vi "Condition _string_4_REJECTION.vi"(0 "From Date":timestamp format="%<%Y-%m-%d>T", 1 "Select Stakeholder":string(combo), 5 "To Date":timestamp format="%<%Y-%m-%d>T", 7 "Shift":string(combo)="ALL", 9 "Select Station":string(combo)="ST 1", 11 "STACKHOLDER_ID":i32, 12 "Refnum out 2":T1) -> (3 "Array":string[](array[string]), 4 "sum":i32[](array[numeric]), 6 "all station":string[][](array[string]), 8 "Table":string[][](array[string]), 10 "Elements Found out":string[](array[string]), 13 "PROD_COUNT TEST":string[](array[string]), 14 "Refnum out":T1, 15 "Array 3":string[][](array[string]))   [LabVIEW 2017]
uses:
  <vilib>/addons/database/Connection.llb/Conn ObjectReference.ctl
  <vilib>/addons/database/NI_Database_API.lvlib
panel:
  out "COUNT":string[](array[string])
  out "DATE":string[](array[string])
  out "error out":errorcluster
  in  "error in (no error)":errorcluster
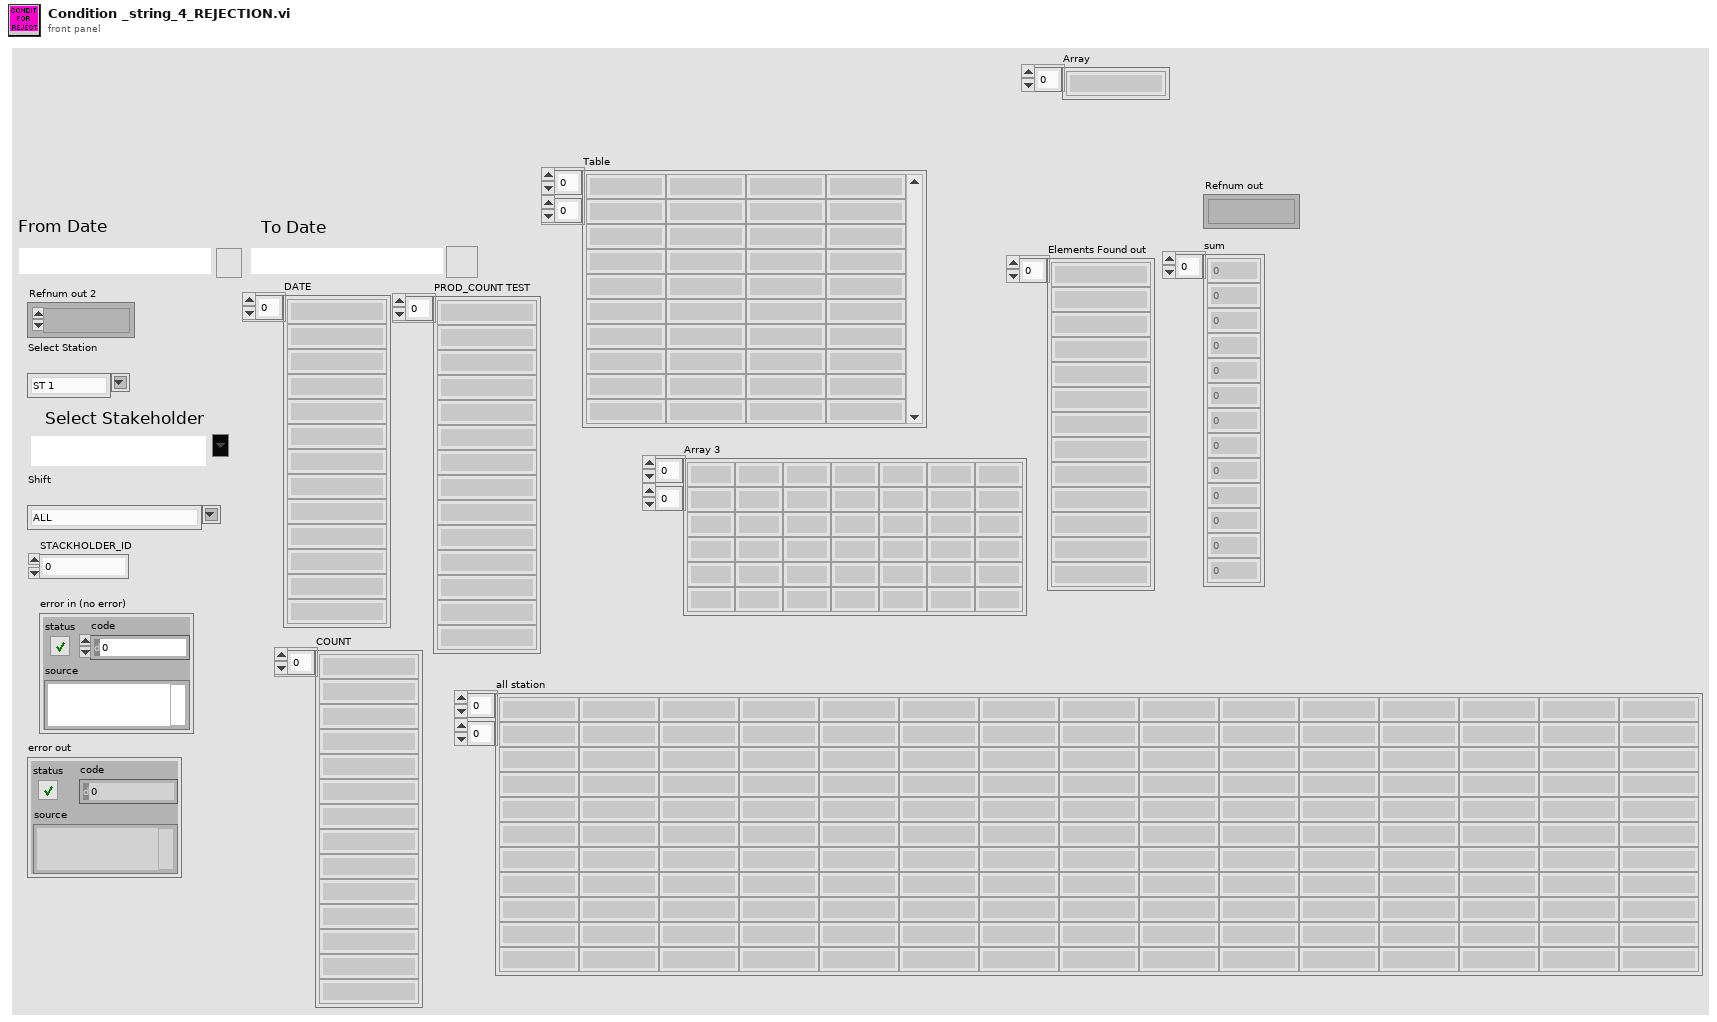
[diagram p1: front panel]
types:
  T1 = typedef "NI_Database_API.lvlib/Conn ObjectReference.ctl" = refnum<k1>
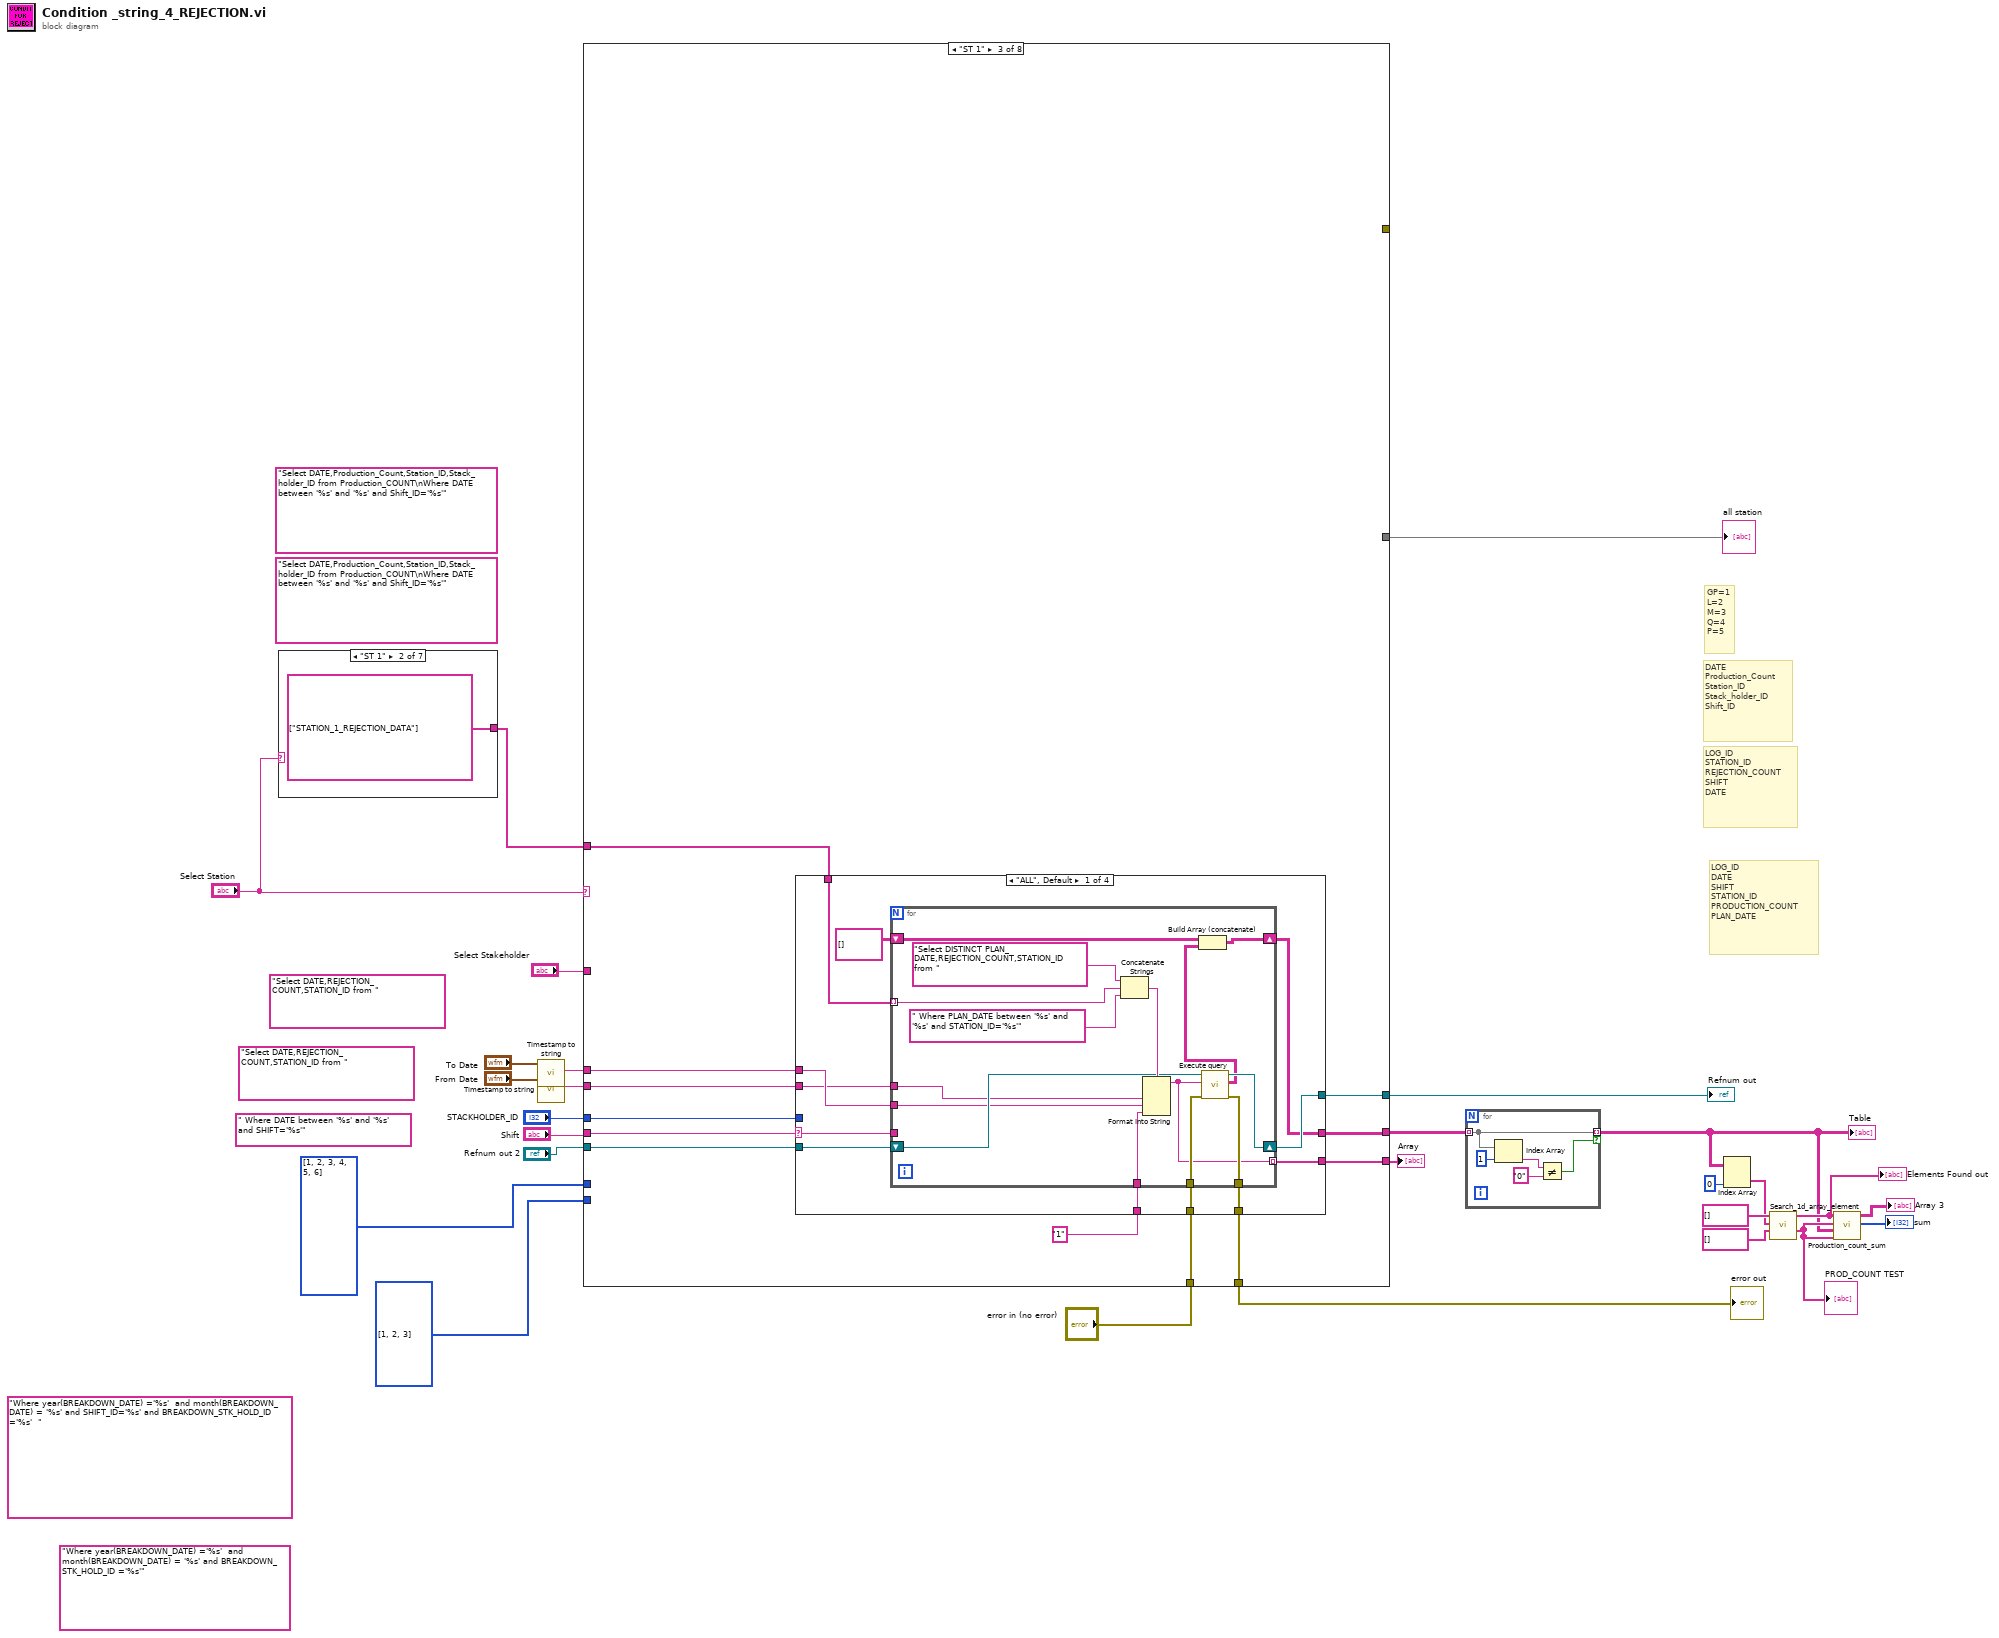
[diagram p0: block diagram]
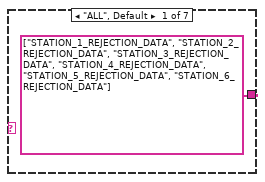
[diagram p2: hidden frame]
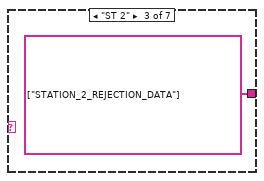
[diagram p3: hidden frame]
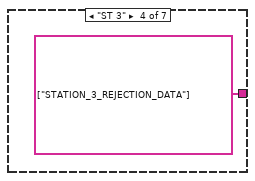
[diagram p4: hidden frame]
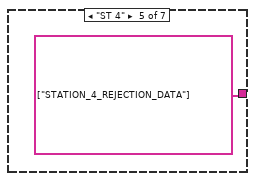
[diagram p5: hidden frame]
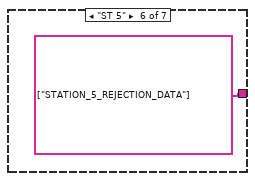
[diagram p6: hidden frame]
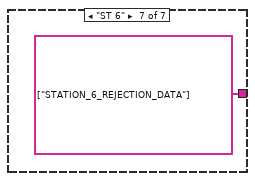
[diagram p7: hidden frame]
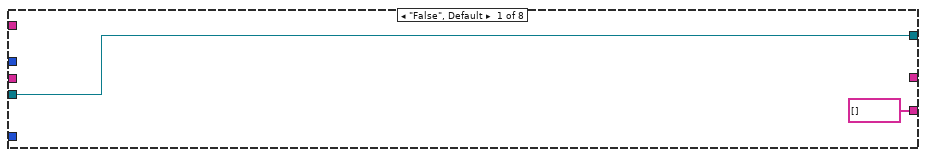
[diagram p8: hidden frame]
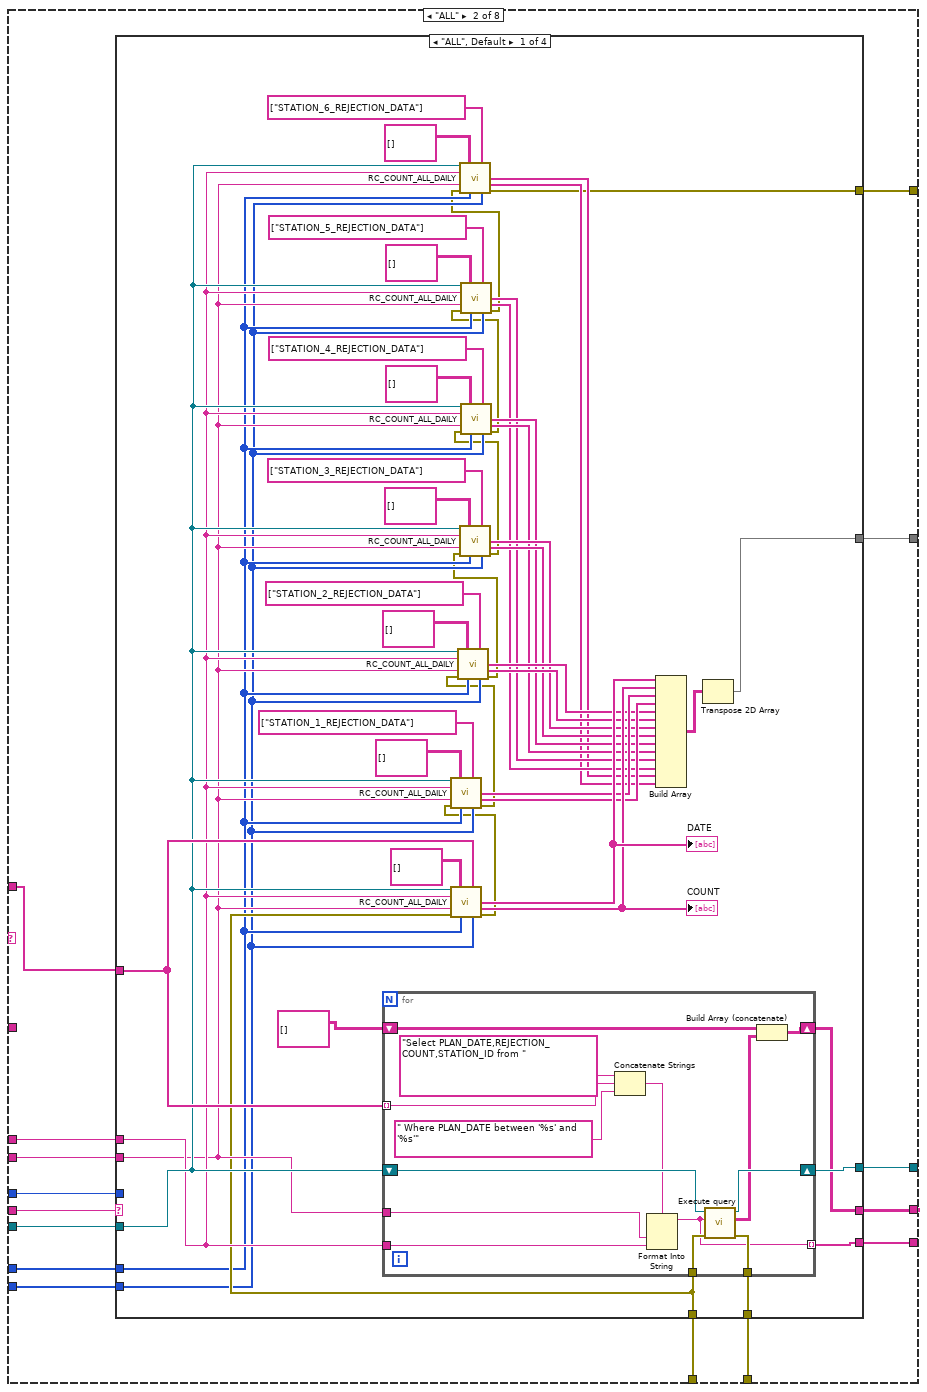
[diagram p9: hidden frame]
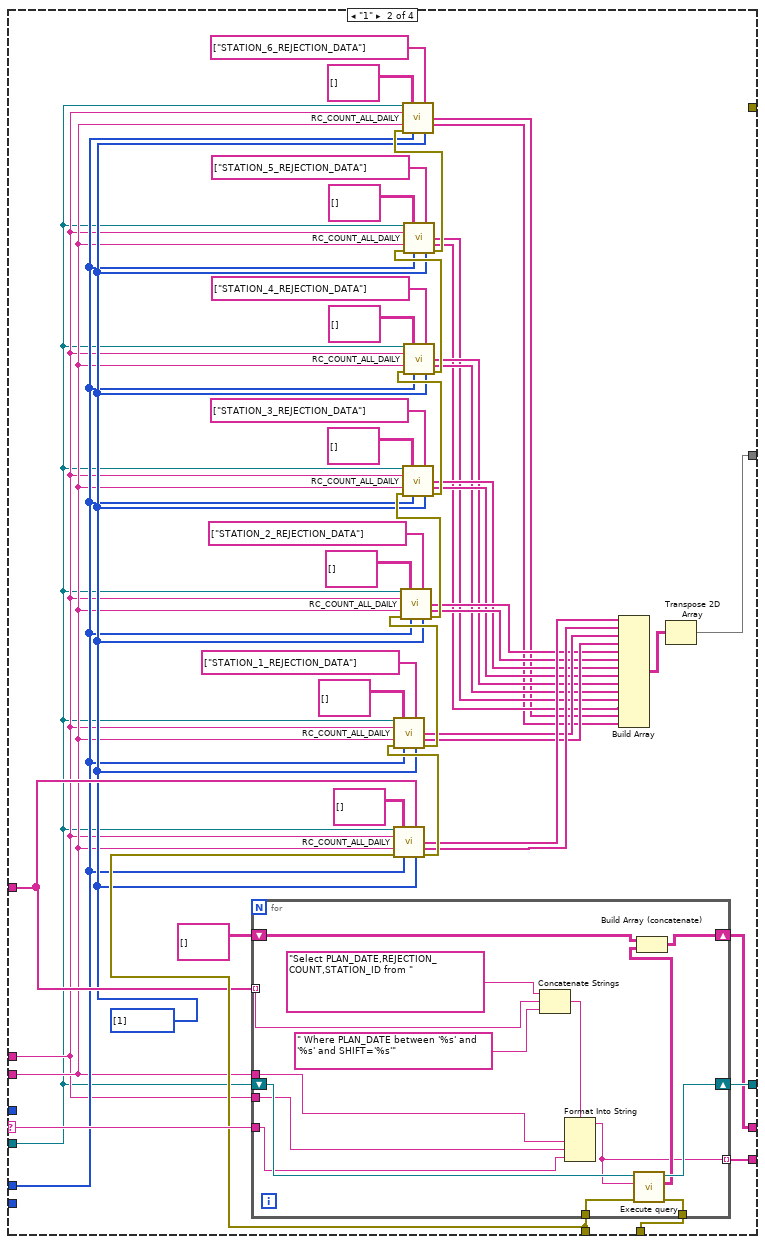
[diagram p10: hidden frame]
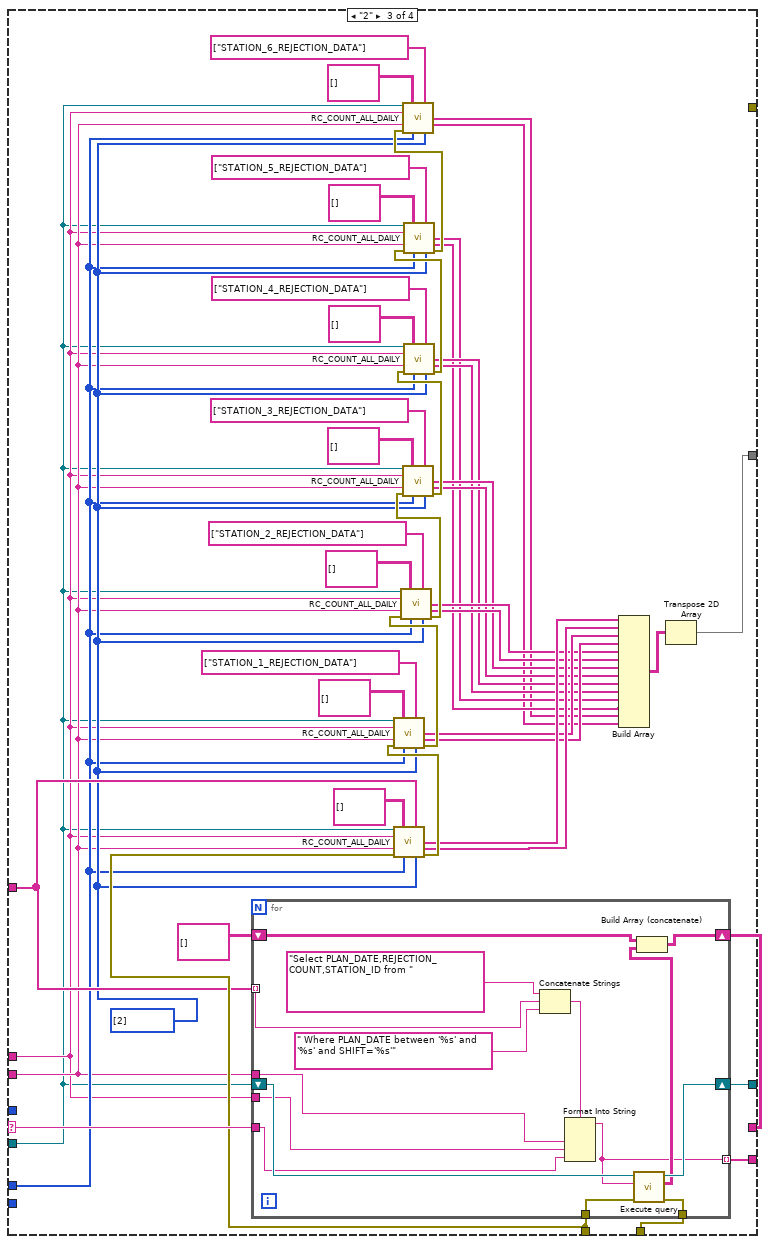
[diagram p11: hidden frame]
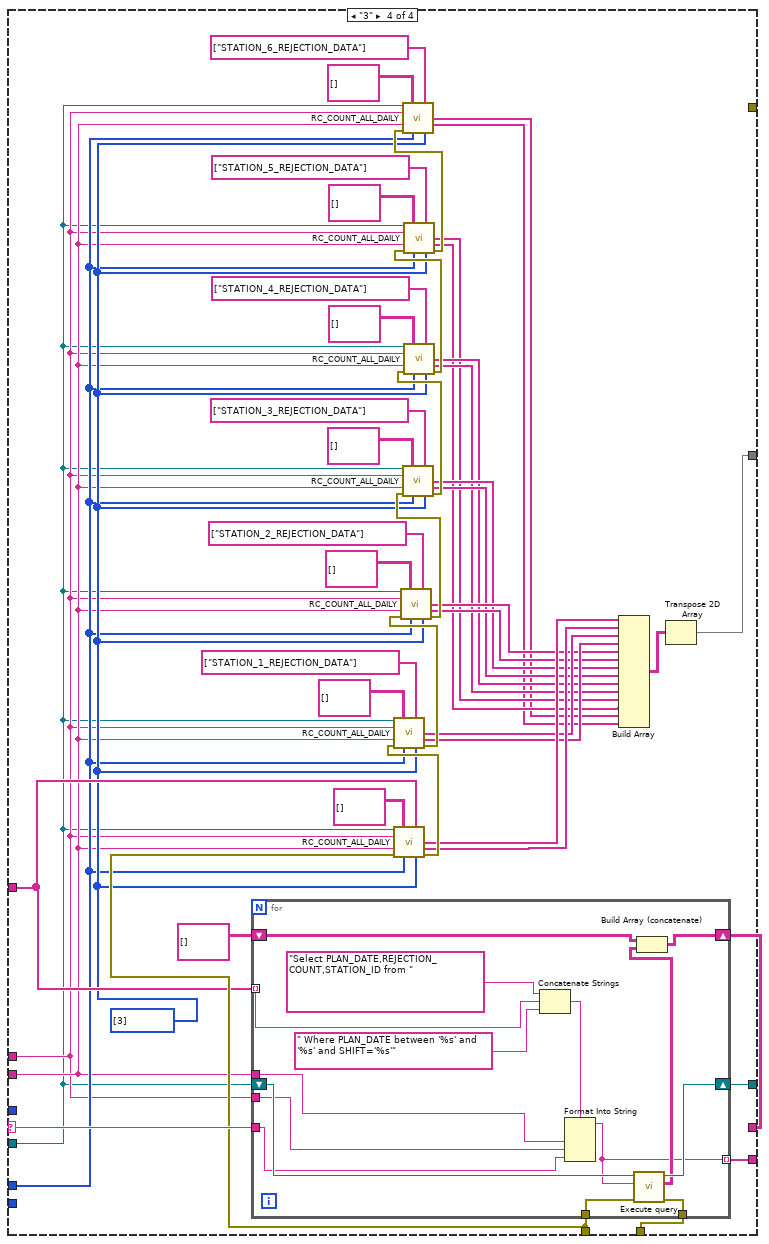
[diagram p12: hidden frame]
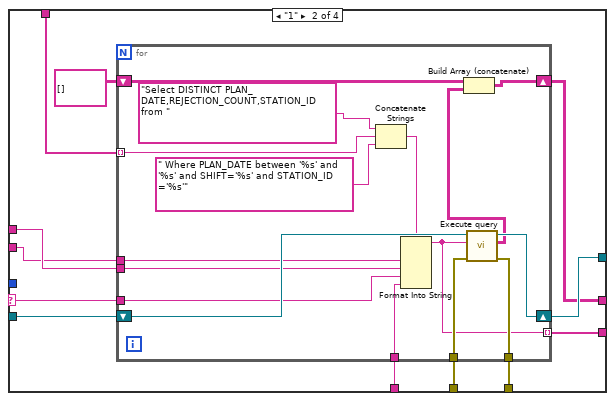
[diagram p13: hidden frame]
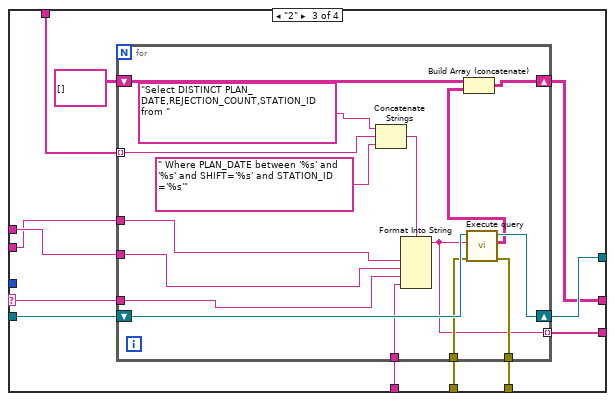
[diagram p14: hidden frame]
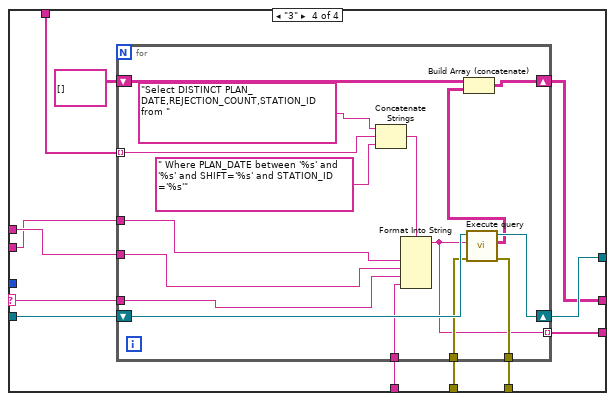
[diagram p15: hidden frame]
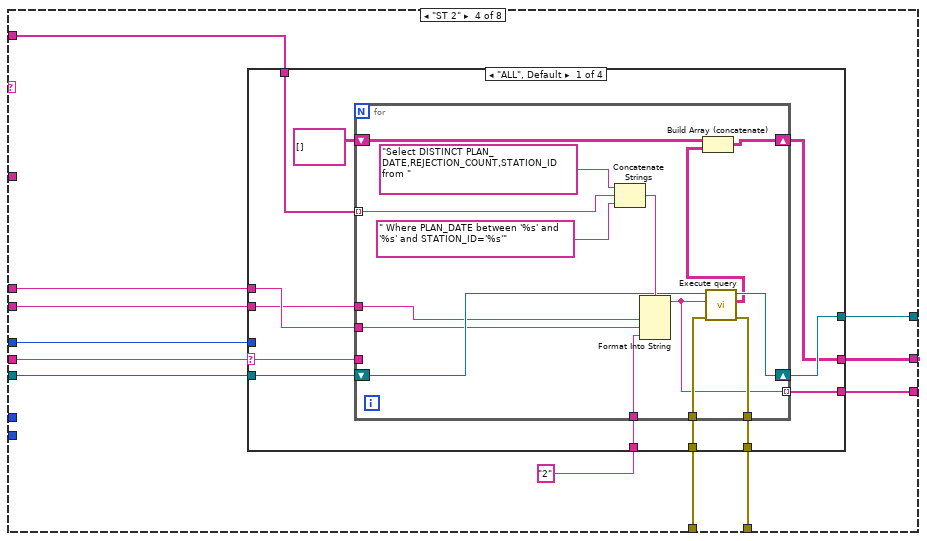
[diagram p16: hidden frame]
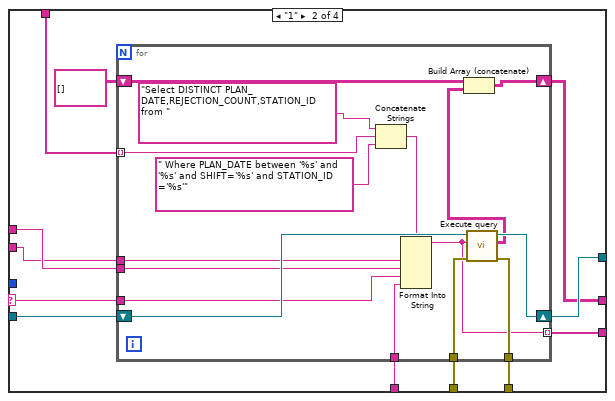
[diagram p17: hidden frame]
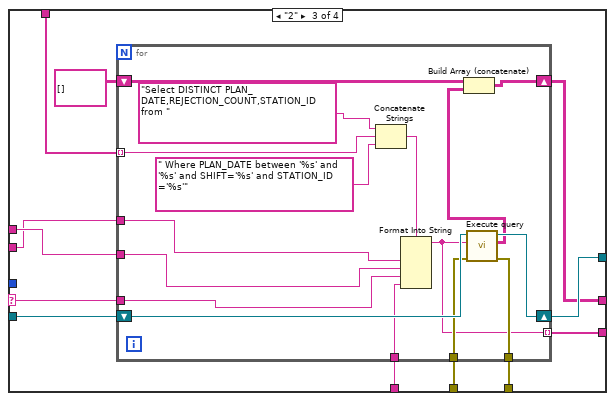
[diagram p18: hidden frame]
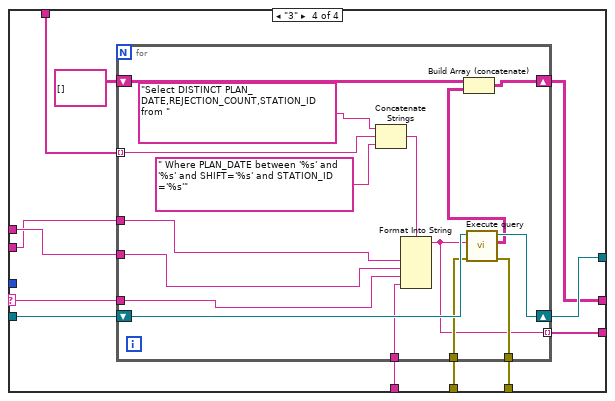
[diagram p19: hidden frame]
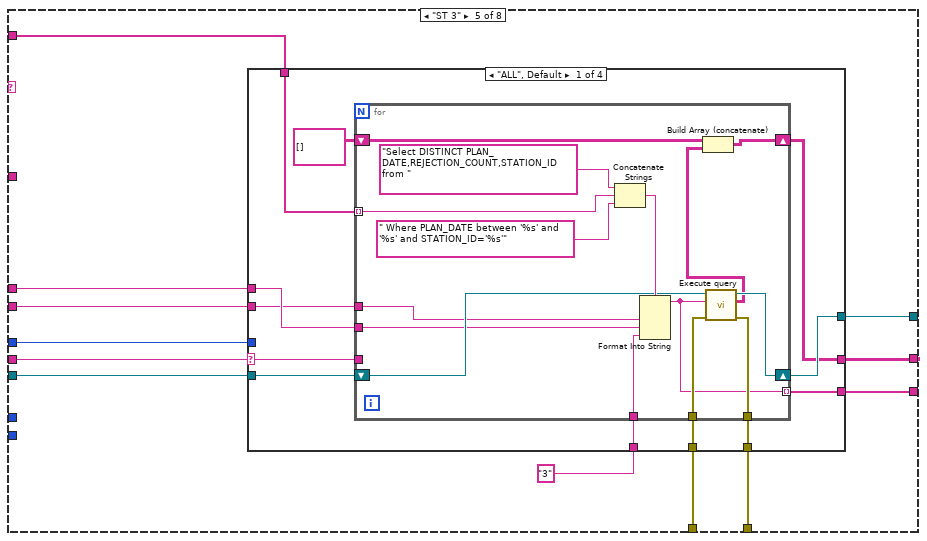
[diagram p20: hidden frame]
diagram:
  (unwired) "Select DATE,REJECTION_COUNT,STATION_ID from "
  (unwired) " Where DATE between '%s' and '%s' and SHIFT='%s'"
  (unwired) "Select DATE,REJECTION_COUNT,STATION_ID from "
  (unwired) "Select DATE,Production_Count,Station_ID,Stack_holder_ID from Production_COUNT\nWhere DATE between '%s' and '%s' and Shift_ID='%s'" ("string")
  (unwired) "Select DATE,Production_Count,Station_ID,Stack_holder_ID from Production_COUNT\nWhere DATE between '%s' and '%s' and Shift_ID='%s'" ("string")
  (unwired) "Where year(BREAKDOWN_DATE) ='%s'  and month(BREAKDOWN_DATE) = '%s' and BREAKDOWN_STK_HOLD_ID ='%s'" ("condition")
  (unwired) "Where year(BREAKDOWN_DATE) ='%s'  and month(BREAKDOWN_DATE) = '%s' and SHIFT_ID='%s' and BREAKDOWN_STK_HOLD_ID ='%s'  " ("condition")
  # "LOG_ID\nSTATION_ID\nREJECTION_COUNT\nSHIFT\nDATE"
  # "LOG_ID\nDATE\nSHIFT\nSTATION_ID\nPRODUCTION_COUNT\nPLAN_DATE"
  # "GP=1\nL=2\nM=3\nQ=4\nP=5"
  # "DATE\nProduction_Count\nStation_ID\nStack_holder_ID\nShift_ID"
  n1 = case shown="\"ST 1\"" "Select Station" {
    tunnel: [string[] ["STATION_1_REJECTION_DATA", "STATION_2_REJECTION_DATA", "STATION_3_REJECTION_DATA", "STATION_4_REJECTION_DATA", "STATION_5_REJECTION_DATA", "STATION_6_REJECTION_DATA"] string[] ["STATION_1_REJECTION_DATA"] string[] ["STATION_2_REJECTION_DATA"] string[] ["STATION_3_REJECTION_DATA"] string[] ["STATION_4_REJECTION_DATA"] string[] ["STATION_5_REJECTION_DATA"] string[] ["STATION_6_REJECTION_DATA"]] -> w14
    frame "ALL", Default {
    }
    frame "ST 1" {
    }
    frame "ST 2" {
    }
    frame "ST 3" {
    }
    frame "ST 4" {
    }
    frame "ST 5" {
    }
    frame "ST 6" {
    }
  }
  n2 = call "Timestamp to string.vi"("time stamp"="To Date") -> ("Date"=w6:string)  [unwired: 8 in, 2 out]
  n3 = call "Timestamp to string.vi"("time stamp"="From Date") -> ("Date"=w4:string)  [unwired: 8 in, 2 out]
  n4 = case shown="\"ST 1\"" "Select Station" {
    tunnel: "Shift" -> [_ w51 w314 w437 w560 w683 w806 w929]
    tunnel: w6 -> [_ w50 w313 w436 w559 w682 w805 w928]
    tunnel: w4 -> [_ w49 w312 w435 w558 w681 w804 w927]
    tunnel: "STACKHOLDER_ID" -> [_ w48 w311 w434 w557 w680 w803 w926]
    tunnel: [_ w47 w310 w433 w556 w679 w802 w925] -> w2
    tunnel: "Refnum out 2" -> [w36 w46 w309 w432 w555 w678 w801 w924]
    tunnel: [w36 w45 w308 w431 w554 w677 w800 w923] -> w24
    tunnel: "Select Stakeholder" -> [_ _ _ _ _ _ _ _]
    tunnel: w14 -> [_ w44 w307 w430 w553 w676 w799 w922]
    tunnel: "error in (no error)" -> [_ w43 w306 w429 w552 w675 w798 w921]
    tunnel: [_ w42 w305 w428 w551 w674 w797 w920] -> w12
    tunnel: i32[] [1, 2, 3, 4, 5, 6] -> [_ w41 _ _ _ _ _ _]
    tunnel: i32[] [1, 2, 3] -> [_ w40 _ _ _ _ _ _]
    tunnel: [_ w39 _ _ _ _ _ _] -> w8
    tunnel: [_ w38 _ _ _ _ _ _] -> _
    tunnel: [string[] [] w37 w303 w426 w549 w672 w795 w918] -> w3
    frame "False", Default {
    }
    frame "ALL" {
      n5 = case shown="\"ALL\", Default" w51 {
        selector: w51 -> [_ w160 w223 w286]
        tunnel: w50 -> [w69 w132 w195 w258]
        tunnel: w49 -> [w68 w133 w196 w259]
        tunnel: w48 -> [_ _ _ _]
        tunnel: [w97 w158 w221 w284] -> w47
        tunnel: w46 -> [w70 w131 w194 w257]
        tunnel: [w99 w161 w224 w287] -> w45
        tunnel: w44 -> [w95 w136 w199 w262]
        tunnel: w43 -> [w67 w137 w200 w263]
        tunnel: [w96 w157 w220 w283] -> w42
        tunnel: w41 -> [w66 w134 w197 w260]
        tunnel: w40 -> [w65 _ _ _]
        tunnel: [w60 w115 w178 w241] -> w39
        tunnel: [w53 _ _ _] -> w38
        tunnel: [w52 w114 w177 w240] -> w37
        frame "ALL", Default {
          n6 = for {
            tunnel: w69 -> [w101]
            tunnel: w68 -> [w102]
            shift-right: [w112] -> w99
            shift-left: w70 -> [w113]
            tunnel: w95 -> [w111] mode=indexing
            shift-right: [w106] -> w97
            shift-left: string[][] [] ("data") -> [w108]
            tunnel: w67 -> [w104]
            tunnel: [w103] -> w96
            tunnel: [w100] -> w52 mode=indexing
            n7 = Concatenate Strings("Select PLAN_DATE,REJECTION_COUNT,STATION_ID from ", w111, " Where PLAN_DATE between '%s' and '%s'") -> (w109:string)
            n8 = Format Into String(format string=w109, w102, w101) -> (resulting string=w100:string)  [unwired: 2 in, 1 out]
            n9 = call "Execute query.vi"("error in (no error)"=w104, "String"=w100, "connection reference"=w113) -> ("error out"=w103:errorcluster, "Table"=w107:string[][], "connection reference 2"=w112:T1)  [unwired: 3 in, 3 out]
            n10 = Build Array (concatenate)(w108, w107) -> (w106:string[][])
          }
          n11 = call "RC_COUNT_ALL_DAILY.vi"("Refnum in"=w70, "data in"=string[][] [] ("data"), "Array 3"=w95, "To Date"=w69, "From Date"=w68, "error in (no error)"=w67, "STATION"=w66, "SHIFT"=w65) -> ("DATE"=w91:string[], "COUNT"=w90:string[], "error out"=w59:errorcluster)  [unwired: 3 in, 2 out]
          "DATE" <- w91
          "COUNT" <- w90
          n12 = call "RC_COUNT_ALL_DAILY.vi"("Refnum in"=w70, "data in"=string[][] [] ("data"), "Array 3"=string[] ["STATION_1_REJECTION_DATA"], "To Date"=w69, "From Date"=w68, "error in (no error)"=w59, "STATION"=w66, "SHIFT"=w65) -> ("DATE"=w89:string[], "COUNT"=w88:string[], "error out"=w58:errorcluster)  [unwired: 3 in, 2 out]
          n13 = call "RC_COUNT_ALL_DAILY.vi"("Refnum in"=w70, "data in"=string[][] [] ("data"), "Array 3"=string[] ["STATION_2_REJECTION_DATA"], "To Date"=w69, "From Date"=w68, "error in (no error)"=w58, "STATION"=w66, "SHIFT"=w65) -> ("DATE"=w84:string[], "COUNT"=w83:string[], "error out"=w57:errorcluster)  [unwired: 3 in, 2 out]
          n14 = call "RC_COUNT_ALL_DAILY.vi"("Refnum in"=w70, "data in"=string[][] [] ("data"), "Array 3"=string[] ["STATION_3_REJECTION_DATA"], "To Date"=w69, "From Date"=w68, "error in (no error)"=w57, "STATION"=w66, "SHIFT"=w65) -> ("DATE"=w80:string[], "COUNT"=w79:string[], "error out"=w56:errorcluster)  [unwired: 3 in, 2 out]
          n15 = call "RC_COUNT_ALL_DAILY.vi"("Refnum in"=w70, "data in"=string[][] [] ("data"), "Array 3"=string[] ["STATION_4_REJECTION_DATA"], "To Date"=w69, "From Date"=w68, "error in (no error)"=w56, "STATION"=w66, "SHIFT"=w65) -> ("DATE"=w76:string[], "COUNT"=w75:string[], "error out"=w55:errorcluster)  [unwired: 3 in, 2 out]
          n16 = call "RC_COUNT_ALL_DAILY.vi"("Refnum in"=w70, "data in"=string[][] [] ("data"), "Array 3"=string[] ["STATION_5_REJECTION_DATA"], "To Date"=w69, "From Date"=w68, "error in (no error)"=w55, "STATION"=w66, "SHIFT"=w65) -> ("DATE"=w64:string[], "COUNT"=w63:string[], "error out"=w54:errorcluster)  [unwired: 3 in, 2 out]
          n17 = call "RC_COUNT_ALL_DAILY.vi"("Refnum in"=w70, "data in"=string[][] [] ("data"), "Array 3"=string[] ["STATION_6_REJECTION_DATA"], "To Date"=w69, "From Date"=w68, "error in (no error)"=w54, "STATION"=w66, "SHIFT"=w65) -> ("DATE"=w62:string[], "COUNT"=w61:string[], "error out"=w53:errorcluster)  [unwired: 3 in, 2 out]
          n18 = Build Array(w91, w90, w89, w88, w84, w83, w80, w79, w76, w75, w64, w63, w62, w61) -> (w87:string[][])
          n19 = Transpose 2D Array(2D array=w87) -> (transposed array=w60:string[][])
        }
        frame "1" {
          w135 = i32[] [1]
          n20 = for {
            tunnel: w132 -> [w163]
            tunnel: w133 -> [w164]
            tunnel: w160 -> [w174]
            shift-right: [w175] -> w161
            shift-left: w131 -> [w176]
            tunnel: w136 -> [w172] mode=indexing
            shift-right: [w169] -> w158
            shift-left: string[][] [] ("data") -> [w170]
            tunnel: w137 -> [w167]
            tunnel: [w166] -> w157
            tunnel: [w162] -> w114 mode=indexing
            n21 = Concatenate Strings("Select PLAN_DATE,REJECTION_COUNT,STATION_ID from ", w172, " Where PLAN_DATE between '%s' and '%s' and SHIFT='%s'") -> (w173:string)
            n22 = Format Into String(format string=w173, w164, w163, w174) -> (resulting string=w162:string)  [unwired: 2 in, 1 out]
            n23 = call "Execute query.vi"("error in (no error)"=w167, "String"=w162, "connection reference"=w176) -> ("error out"=w166:errorcluster, "Table"=w168:string[][], "connection reference 2"=w175:T1)  [unwired: 3 in, 3 out]
            n24 = Build Array (concatenate)(w170, w168) -> (w169:string[][])
          }
          n25 = call "RC_COUNT_ALL_DAILY.vi"("Refnum in"=w131, "data in"=string[][] [] ("data"), "Array 3"=w136, "To Date"=w132, "From Date"=w133, "error in (no error)"=w137, "STATION"=w134, "SHIFT"=w135) -> ("DATE"=w129:string[], "COUNT"=w128:string[], "error out"=w143:errorcluster)  [unwired: 3 in, 2 out]
          n26 = call "RC_COUNT_ALL_DAILY.vi"("Refnum in"=w131, "data in"=string[][] [] ("data"), "Array 3"=string[] ["STATION_1_REJECTION_DATA"], "To Date"=w132, "From Date"=w133, "error in (no error)"=w143, "STATION"=w134, "SHIFT"=w135) -> ("DATE"=w127:string[], "COUNT"=w126:string[], "error out"=w142:errorcluster)  [unwired: 3 in, 2 out]
          n27 = call "RC_COUNT_ALL_DAILY.vi"("Refnum in"=w131, "data in"=string[][] [] ("data"), "Array 3"=string[] ["STATION_2_REJECTION_DATA"], "To Date"=w132, "From Date"=w133, "error in (no error)"=w142, "STATION"=w134, "SHIFT"=w135) -> ("DATE"=w125:string[], "COUNT"=w124:string[], "error out"=w141:errorcluster)  [unwired: 3 in, 2 out]
          n28 = call "RC_COUNT_ALL_DAILY.vi"("Refnum in"=w131, "data in"=string[][] [] ("data"), "Array 3"=string[] ["STATION_3_REJECTION_DATA"], "To Date"=w132, "From Date"=w133, "error in (no error)"=w141, "STATION"=w134, "SHIFT"=w135) -> ("DATE"=w123:string[], "COUNT"=w122:string[], "error out"=w140:errorcluster)  [unwired: 3 in, 2 out]
          n29 = call "RC_COUNT_ALL_DAILY.vi"("Refnum in"=w131, "data in"=string[][] [] ("data"), "Array 3"=string[] ["STATION_4_REJECTION_DATA"], "To Date"=w132, "From Date"=w133, "error in (no error)"=w140, "STATION"=w134, "SHIFT"=w135) -> ("DATE"=w121:string[], "COUNT"=w120:string[], "error out"=w139:errorcluster)  [unwired: 3 in, 2 out]
          n30 = call "RC_COUNT_ALL_DAILY.vi"("Refnum in"=w131, "data in"=string[][] [] ("data"), "Array 3"=string[] ["STATION_5_REJECTION_DATA"], "To Date"=w132, "From Date"=w133, "error in (no error)"=w139, "STATION"=w134, "SHIFT"=w135) -> ("DATE"=w119:string[], "COUNT"=w118:string[], "error out"=w138:errorcluster)  [unwired: 3 in, 2 out]
          n31 = call "RC_COUNT_ALL_DAILY.vi"("Refnum in"=w131, "data in"=string[][] [] ("data"), "Array 3"=string[] ["STATION_6_REJECTION_DATA"], "To Date"=w132, "From Date"=w133, "error in (no error)"=w138, "STATION"=w134, "SHIFT"=w135) -> ("DATE"=w117:string[], "COUNT"=w116:string[])  [unwired: 3 in, 3 out]
          n32 = Build Array(w129, w128, w127, w126, w125, w124, w123, w122, w121, w120, w119, w118, w117, w116) -> (w130:string[][])
          n33 = Transpose 2D Array(2D array=w130) -> (transposed array=w115:string[][])
        }
        frame "2" {
          w198 = i32[] [2]
          n34 = for {
            tunnel: w195 -> [w226]
            tunnel: w196 -> [w227]
            tunnel: w223 -> [w237]
            shift-right: [w238] -> w224
            shift-left: w194 -> [w239]
            tunnel: w199 -> [w235] mode=indexing
            shift-right: [w232] -> w221
            shift-left: string[][] [] ("data") -> [w233]
            tunnel: w200 -> [w230]
            tunnel: [w229] -> w220
            tunnel: [w225] -> w177 mode=indexing
            n35 = Concatenate Strings("Select PLAN_DATE,REJECTION_COUNT,STATION_ID from ", w235, " Where PLAN_DATE between '%s' and '%s' and SHIFT='%s'") -> (w236:string)
            n36 = Format Into String(format string=w236, w227, w226, w237) -> (resulting string=w225:string)  [unwired: 2 in, 1 out]
            n37 = call "Execute query.vi"("error in (no error)"=w230, "String"=w225, "connection reference"=w239) -> ("error out"=w229:errorcluster, "Table"=w231:string[][], "connection reference 2"=w238:T1)  [unwired: 3 in, 3 out]
            n38 = Build Array (concatenate)(w233, w231) -> (w232:string[][])
          }
          n39 = call "RC_COUNT_ALL_DAILY.vi"("Refnum in"=w194, "data in"=string[][] [] ("data"), "Array 3"=w199, "To Date"=w195, "From Date"=w196, "error in (no error)"=w200, "STATION"=w197, "SHIFT"=w198) -> ("DATE"=w192:string[], "COUNT"=w191:string[], "error out"=w206:errorcluster)  [unwired: 3 in, 2 out]
          n40 = call "RC_COUNT_ALL_DAILY.vi"("Refnum in"=w194, "data in"=string[][] [] ("data"), "Array 3"=string[] ["STATION_1_REJECTION_DATA"], "To Date"=w195, "From Date"=w196, "error in (no error)"=w206, "STATION"=w197, "SHIFT"=w198) -> ("DATE"=w190:string[], "COUNT"=w189:string[], "error out"=w205:errorcluster)  [unwired: 3 in, 2 out]
          n41 = call "RC_COUNT_ALL_DAILY.vi"("Refnum in"=w194, "data in"=string[][] [] ("data"), "Array 3"=string[] ["STATION_2_REJECTION_DATA"], "To Date"=w195, "From Date"=w196, "error in (no error)"=w205, "STATION"=w197, "SHIFT"=w198) -> ("DATE"=w188:string[], "COUNT"=w187:string[], "error out"=w204:errorcluster)  [unwired: 3 in, 2 out]
          n42 = call "RC_COUNT_ALL_DAILY.vi"("Refnum in"=w194, "data in"=string[][] [] ("data"), "Array 3"=string[] ["STATION_3_REJECTION_DATA"], "To Date"=w195, "From Date"=w196, "error in (no error)"=w204, "STATION"=w197, "SHIFT"=w198) -> ("DATE"=w186:string[], "COUNT"=w185:string[], "error out"=w203:errorcluster)  [unwired: 3 in, 2 out]
          n43 = call "RC_COUNT_ALL_DAILY.vi"("Refnum in"=w194, "data in"=string[][] [] ("data"), "Array 3"=string[] ["STATION_4_REJECTION_DATA"], "To Date"=w195, "From Date"=w196, "error in (no error)"=w203, "STATION"=w197, "SHIFT"=w198) -> ("DATE"=w184:string[], "COUNT"=w183:string[], "error out"=w202:errorcluster)  [unwired: 3 in, 2 out]
          n44 = call "RC_COUNT_ALL_DAILY.vi"("Refnum in"=w194, "data in"=string[][] [] ("data"), "Array 3"=string[] ["STATION_5_REJECTION_DATA"], "To Date"=w195, "From Date"=w196, "error in (no error)"=w202, "STATION"=w197, "SHIFT"=w198) -> ("DATE"=w182:string[], "COUNT"=w181:string[], "error out"=w201:errorcluster)  [unwired: 3 in, 2 out]
          n45 = call "RC_COUNT_ALL_DAILY.vi"("Refnum in"=w194, "data in"=string[][] [] ("data"), "Array 3"=string[] ["STATION_6_REJECTION_DATA"], "To Date"=w195, "From Date"=w196, "error in (no error)"=w201, "STATION"=w197, "SHIFT"=w198) -> ("DATE"=w180:string[], "COUNT"=w179:string[])  [unwired: 3 in, 3 out]
          n46 = Build Array(w192, w191, w190, w189, w188, w187, w186, w185, w184, w183, w182, w181, w180, w179) -> (w193:string[][])
          n47 = Transpose 2D Array(2D array=w193) -> (transposed array=w178:string[][])
        }
        frame "3" {
          w261 = i32[] [3]
          n48 = for {
            tunnel: w258 -> [w289]
            tunnel: w259 -> [w290]
            tunnel: w286 -> [w300]
            shift-right: [w301] -> w287
            shift-left: w257 -> [w302]
            tunnel: w262 -> [w298] mode=indexing
            shift-right: [w295] -> w284
            shift-left: string[][] [] ("data") -> [w296]
            tunnel: w263 -> [w293]
            tunnel: [w292] -> w283
            tunnel: [w288] -> w240 mode=indexing
            n49 = Concatenate Strings("Select PLAN_DATE,REJECTION_COUNT,STATION_ID from ", w298, " Where PLAN_DATE between '%s' and '%s' and SHIFT='%s'") -> (w299:string)
            n50 = Format Into String(format string=w299, w290, w289, w300) -> (resulting string=w288:string)  [unwired: 2 in, 1 out]
            n51 = call "Execute query.vi"("error in (no error)"=w293, "String"=w288, "connection reference"=w302) -> ("error out"=w292:errorcluster, "Table"=w294:string[][], "connection reference 2"=w301:T1)  [unwired: 3 in, 3 out]
            n52 = Build Array (concatenate)(w296, w294) -> (w295:string[][])
          }
          n53 = call "RC_COUNT_ALL_DAILY.vi"("Refnum in"=w257, "data in"=string[][] [] ("data"), "Array 3"=w262, "To Date"=w258, "From Date"=w259, "error in (no error)"=w263, "STATION"=w260, "SHIFT"=w261) -> ("DATE"=w255:string[], "COUNT"=w254:string[], "error out"=w269:errorcluster)  [unwired: 3 in, 2 out]
          n54 = call "RC_COUNT_ALL_DAILY.vi"("Refnum in"=w257, "data in"=string[][] [] ("data"), "Array 3"=string[] ["STATION_1_REJECTION_DATA"], "To Date"=w258, "From Date"=w259, "error in (no error)"=w269, "STATION"=w260, "SHIFT"=w261) -> ("DATE"=w253:string[], "COUNT"=w252:string[], "error out"=w268:errorcluster)  [unwired: 3 in, 2 out]
          n55 = call "RC_COUNT_ALL_DAILY.vi"("Refnum in"=w257, "data in"=string[][] [] ("data"), "Array 3"=string[] ["STATION_2_REJECTION_DATA"], "To Date"=w258, "From Date"=w259, "error in (no error)"=w268, "STATION"=w260, "SHIFT"=w261) -> ("DATE"=w251:string[], "COUNT"=w250:string[], "error out"=w267:errorcluster)  [unwired: 3 in, 2 out]
          n56 = call "RC_COUNT_ALL_DAILY.vi"("Refnum in"=w257, "data in"=string[][] [] ("data"), "Array 3"=string[] ["STATION_3_REJECTION_DATA"], "To Date"=w258, "From Date"=w259, "error in (no error)"=w267, "STATION"=w260, "SHIFT"=w261) -> ("DATE"=w249:string[], "COUNT"=w248:string[], "error out"=w266:errorcluster)  [unwired: 3 in, 2 out]
          n57 = call "RC_COUNT_ALL_DAILY.vi"("Refnum in"=w257, "data in"=string[][] [] ("data"), "Array 3"=string[] ["STATION_4_REJECTION_DATA"], "To Date"=w258, "From Date"=w259, "error in (no error)"=w266, "STATION"=w260, "SHIFT"=w261) -> ("DATE"=w247:string[], "COUNT"=w246:string[], "error out"=w265:errorcluster)  [unwired: 3 in, 2 out]
          n58 = call "RC_COUNT_ALL_DAILY.vi"("Refnum in"=w257, "data in"=string[][] [] ("data"), "Array 3"=string[] ["STATION_5_REJECTION_DATA"], "To Date"=w258, "From Date"=w259, "error in (no error)"=w265, "STATION"=w260, "SHIFT"=w261) -> ("DATE"=w245:string[], "COUNT"=w244:string[], "error out"=w264:errorcluster)  [unwired: 3 in, 2 out]
          n59 = call "RC_COUNT_ALL_DAILY.vi"("Refnum in"=w257, "data in"=string[][] [] ("data"), "Array 3"=string[] ["STATION_6_REJECTION_DATA"], "To Date"=w258, "From Date"=w259, "error in (no error)"=w264, "STATION"=w260, "SHIFT"=w261) -> ("DATE"=w243:string[], "COUNT"=w242:string[])  [unwired: 3 in, 3 out]
          n60 = Build Array(w255, w254, w253, w252, w251, w250, w249, w248, w247, w246, w245, w244, w243, w242) -> (w256:string[][])
          n61 = Transpose 2D Array(2D array=w256) -> (transposed array=w241:string[][])
        }
      }
    }
    frame "ST 1" {
      n62 = case shown="\"ALL\", Default" w314 {
        selector: w314 -> [w322 w349 w377 w405]
        tunnel: w313 -> [w326 w353 w381 w409]
        tunnel: w312 -> [w325 w352 w380 w408]
        tunnel: w311 -> [_ _ _ _]
        tunnel: [w319 w346 w374 w402] -> w310
        tunnel: w309 -> [w324 w351 w379 w407]
        tunnel: [w323 w350 w378 w406] -> w308
        tunnel: w307 -> [w321 w348 w376 w404]
        tunnel: w306 -> [w318 w344 w372 w400]
        tunnel: [w317 w345 w373 w401] -> w305
        tunnel: "1" -> [w316 w343 w371 w399]
        tunnel: [w315 w342 w370 w398] -> w303
        frame "ALL", Default {
          n63 = for {
            tunnel: w326 -> [w329]
            tunnel: w325 -> [w330]
            tunnel: w322 -> [_]
            tunnel: w321 -> [w340] mode=indexing
            shift-right: [w341] -> w323
            shift-left: w324 -> [w335]
            shift-right: [w336] -> w319
            shift-left: string[][] [] ("data") -> [w338]
            tunnel: w318 -> [w334]
            tunnel: [w333] -> w317
            tunnel: w316 -> [w328]
            tunnel: [w327] -> w315 mode=indexing
            n64 = Concatenate Strings("Select DISTINCT PLAN_DATE,REJECTION_COUNT,STATION_ID from ", w340, " Where PLAN_DATE between '%s' and '%s' and STATION_ID='%s'") -> (w339:string)
            n65 = Format Into String(format string=w339, w330, w329, w328) -> (resulting string=w327:string)  [unwired: 2 in, 1 out]
            n66 = call "Execute query.vi"("error in (no error)"=w334, "String"=w327, "connection reference"=w335) -> ("error out"=w333:errorcluster, "Table"=w337:string[][], "connection reference 2"=w341:T1)  [unwired: 3 in, 3 out]
            n67 = Build Array (concatenate)(w338, w337) -> (w336:string[][])
          }
        }
        frame "1" {
          n68 = for {
            tunnel: w353 -> [w356]
            tunnel: w352 -> [w357]
            tunnel: w349 -> [w367]
            tunnel: w348 -> [w366] mode=indexing
            shift-right: [w368] -> w350
            shift-left: w351 -> [w369]
            shift-right: [w361] -> w346
            shift-left: string[][] [] ("data") -> [w363]
            tunnel: [w360] -> w345
            tunnel: w344 -> [w359]
            tunnel: w343 -> [w355]
            tunnel: [w354] -> w342 mode=indexing
            n69 = Concatenate Strings("Select DISTINCT PLAN_DATE,REJECTION_COUNT,STATION_ID from ", w366, " Where PLAN_DATE between '%s' and '%s' and SHIFT='%s' and STATION_ID ='%s'") -> (w364:string)
            n70 = Format Into String(format string=w364, w357, w356, w367, w355) -> (resulting string=w354:string)  [unwired: 2 in, 1 out]
            n71 = call "Execute query.vi"("error in (no error)"=w359, "String"=w354, "connection reference"=w369) -> ("error out"=w360:errorcluster, "Table"=w362:string[][], "connection reference 2"=w368:T1)  [unwired: 3 in, 3 out]
            n72 = Build Array (concatenate)(w363, w362) -> (w361:string[][])
          }
        }
        frame "2" {
          n73 = for {
            tunnel: w381 -> [w384]
            tunnel: w380 -> [w385]
            tunnel: w377 -> [w395]
            tunnel: w376 -> [w394] mode=indexing
            shift-right: [w396] -> w378
            shift-left: w379 -> [w397]
            shift-right: [w389] -> w374
            shift-left: string[][] [] ("data") -> [w391]
            tunnel: [w388] -> w373
            tunnel: w372 -> [w387]
            tunnel: w371 -> [w383]
            tunnel: [w382] -> w370 mode=indexing
            n74 = Concatenate Strings("Select DISTINCT PLAN_DATE,REJECTION_COUNT,STATION_ID from ", w394, " Where PLAN_DATE between '%s' and '%s' and SHIFT='%s' and STATION_ID ='%s'") -> (w392:string)
            n75 = Format Into String(format string=w392, w385, w384, w395, w383) -> (resulting string=w382:string)  [unwired: 2 in, 1 out]
            n76 = call "Execute query.vi"("error in (no error)"=w387, "String"=w382, "connection reference"=w397) -> ("error out"=w388:errorcluster, "Table"=w390:string[][], "connection reference 2"=w396:T1)  [unwired: 3 in, 3 out]
            n77 = Build Array (concatenate)(w391, w390) -> (w389:string[][])
          }
        }
        frame "3" {
          n78 = for {
            tunnel: w409 -> [w412]
            tunnel: w408 -> [w413]
            tunnel: w405 -> [w423]
            tunnel: w404 -> [w422] mode=indexing
            shift-right: [w424] -> w406
            shift-left: w407 -> [w425]
            shift-right: [w417] -> w402
            shift-left: string[][] [] ("data") -> [w419]
            tunnel: [w416] -> w401
            tunnel: w400 -> [w415]
            tunnel: w399 -> [w411]
            tunnel: [w410] -> w398 mode=indexing
            n79 = Concatenate Strings("Select DISTINCT PLAN_DATE,REJECTION_COUNT,STATION_ID from ", w422, " Where PLAN_DATE between '%s' and '%s' and SHIFT='%s' and STATION_ID ='%s'") -> (w420:string)
            n80 = Format Into String(format string=w420, w413, w412, w423, w411) -> (resulting string=w410:string)  [unwired: 2 in, 1 out]
            n81 = call "Execute query.vi"("error in (no error)"=w415, "String"=w410, "connection reference"=w425) -> ("error out"=w416:errorcluster, "Table"=w418:string[][], "connection reference 2"=w424:T1)  [unwired: 3 in, 3 out]
            n82 = Build Array (concatenate)(w419, w418) -> (w417:string[][])
          }
        }
      }
    }
    frame "ST 2" {
      n83 = case shown="\"ALL\", Default" w437 {
        selector: w437 -> [w445 w472 w500 w528]
        tunnel: w436 -> [w449 w476 w504 w532]
        tunnel: w435 -> [w448 w475 w503 w531]
        tunnel: w434 -> [_ _ _ _]
        tunnel: [w442 w469 w497 w525] -> w433
        tunnel: w432 -> [w447 w474 w502 w530]
        tunnel: [w446 w473 w501 w529] -> w431
        tunnel: w430 -> [w444 w471 w499 w527]
        tunnel: w429 -> [w441 w467 w495 w523]
        tunnel: [w440 w468 w496 w524] -> w428
        tunnel: "2" -> [w439 w466 w494 w522]
        tunnel: [w438 w465 w493 w521] -> w426
        frame "ALL", Default {
          n84 = for {
            tunnel: w449 -> [w452]
            tunnel: w448 -> [w453]
            tunnel: w445 -> [_]
            tunnel: w444 -> [w463] mode=indexing
            shift-right: [w464] -> w446
            shift-left: w447 -> [w458]
            shift-right: [w459] -> w442
            shift-left: string[][] [] ("data") -> [w461]
            tunnel: w441 -> [w457]
            tunnel: [w456] -> w440
            tunnel: w439 -> [w451]
            tunnel: [w450] -> w438 mode=indexing
            n85 = Concatenate Strings("Select DISTINCT PLAN_DATE,REJECTION_COUNT,STATION_ID from ", w463, " Where PLAN_DATE between '%s' and '%s' and STATION_ID='%s'") -> (w462:string)
            n86 = Format Into String(format string=w462, w453, w452, w451) -> (resulting string=w450:string)  [unwired: 2 in, 1 out]
            n87 = call "Execute query.vi"("error in (no error)"=w457, "String"=w450, "connection reference"=w458) -> ("error out"=w456:errorcluster, "Table"=w460:string[][], "connection reference 2"=w464:T1)  [unwired: 3 in, 3 out]
            n88 = Build Array (concatenate)(w461, w460) -> (w459:string[][])
          }
        }
        frame "1" {
          n89 = for {
            tunnel: w476 -> [w479]
            tunnel: w475 -> [w480]
            tunnel: w472 -> [w490]
            tunnel: w471 -> [w489] mode=indexing
            shift-right: [w491] -> w473
            shift-left: w474 -> [w492]
            shift-right: [w484] -> w469
            shift-left: string[][] [] ("data") -> [w486]
            tunnel: [w483] -> w468
            tunnel: w467 -> [w482]
            tunnel: w466 -> [w478]
            tunnel: [w477] -> w465 mode=indexing
            n90 = Concatenate Strings("Select DISTINCT PLAN_DATE,REJECTION_COUNT,STATION_ID from ", w489, " Where PLAN_DATE between '%s' and '%s' and SHIFT='%s' and STATION_ID ='%s'") -> (w487:string)
            n91 = Format Into String(format string=w487, w480, w479, w490, w478) -> (resulting string=w477:string)  [unwired: 2 in, 1 out]
            n92 = call "Execute query.vi"("error in (no error)"=w482, "String"=w477, "connection reference"=w492) -> ("error out"=w483:errorcluster, "Table"=w485:string[][], "connection reference 2"=w491:T1)  [unwired: 3 in, 3 out]
            n93 = Build Array (concatenate)(w486, w485) -> (w484:string[][])
          }
        }
        frame "2" {
          n94 = for {
            tunnel: w504 -> [w507]
            tunnel: w503 -> [w508]
            tunnel: w500 -> [w518]
            tunnel: w499 -> [w517] mode=indexing
            shift-right: [w519] -> w501
            shift-left: w502 -> [w520]
            shift-right: [w512] -> w497
            shift-left: string[][] [] ("data") -> [w514]
            tunnel: [w511] -> w496
            tunnel: w495 -> [w510]
            tunnel: w494 -> [w506]
            tunnel: [w505] -> w493 mode=indexing
            n95 = Concatenate Strings("Select DISTINCT PLAN_DATE,REJECTION_COUNT,STATION_ID from ", w517, " Where PLAN_DATE between '%s' and '%s' and SHIFT='%s' and STATION_ID ='%s'") -> (w515:string)
            n96 = Format Into String(format string=w515, w508, w507, w518, w506) -> (resulting string=w505:string)  [unwired: 2 in, 1 out]
            n97 = call "Execute query.vi"("error in (no error)"=w510, "String"=w505, "connection reference"=w520) -> ("error out"=w511:errorcluster, "Table"=w513:string[][], "connection reference 2"=w519:T1)  [unwired: 3 in, 3 out]
            n98 = Build Array (concatenate)(w514, w513) -> (w512:string[][])
          }
        }
        frame "3" {
          n99 = for {
            tunnel: w532 -> [w535]
            tunnel: w531 -> [w536]
            tunnel: w528 -> [w546]
            tunnel: w527 -> [w545] mode=indexing
            shift-right: [w547] -> w529
            shift-left: w530 -> [w548]
            shift-right: [w540] -> w525
            shift-left: string[][] [] ("data") -> [w542]
            tunnel: [w539] -> w524
            tunnel: w523 -> [w538]
            tunnel: w522 -> [w534]
            tunnel: [w533] -> w521 mode=indexing
            n100 = Concatenate Strings("Select DISTINCT PLAN_DATE,REJECTION_COUNT,STATION_ID from ", w545, " Where PLAN_DATE between '%s' and '%s' and SHIFT='%s' and STATION_ID ='%s'") -> (w543:string)
            n101 = Format Into String(format string=w543, w536, w535, w546, w534) -> (resulting string=w533:string)  [unwired: 2 in, 1 out]
            n102 = call "Execute query.vi"("error in (no error)"=w538, "String"=w533, "connection reference"=w548) -> ("error out"=w539:errorcluster, "Table"=w541:string[][], "connection reference 2"=w547:T1)  [unwired: 3 in, 3 out]
            n103 = Build Array (concatenate)(w542, w541) -> (w540:string[][])
          }
        }
      }
    }
    frame "ST 3" {
      n104 = case shown="\"ALL\", Default" w560 {
        selector: w560 -> [w568 w595 w623 w651]
        tunnel: w559 -> [w572 w599 w627 w655]
        tunnel: w558 -> [w571 w598 w626 w654]
        tunnel: w557 -> [_ _ _ _]
        tunnel: [w565 w592 w620 w648] -> w556
        tunnel: w555 -> [w570 w597 w625 w653]
        tunnel: [w569 w596 w624 w652] -> w554
        tunnel: w553 -> [w567 w594 w622 w650]
        tunnel: w552 -> [w564 w590 w618 w646]
        tunnel: [w563 w591 w619 w647] -> w551
        tunnel: "3" -> [w562 w589 w617 w645]
        tunnel: [w561 w588 w616 w644] -> w549
        frame "ALL", Default {
          n105 = for {
            tunnel: w572 -> [w575]
            tunnel: w571 -> [w576]
            tunnel: w568 -> [_]
            tunnel: w567 -> [w586] mode=indexing
            shift-right: [w587] -> w569
            shift-left: w570 -> [w581]
            shift-right: [w582] -> w565
            shift-left: string[][] [] ("data") -> [w584]
            tunnel: w564 -> [w580]
            tunnel: [w579] -> w563
            tunnel: w562 -> [w574]
            tunnel: [w573] -> w561 mode=indexing
            n106 = Concatenate Strings("Select DISTINCT PLAN_DATE,REJECTION_COUNT,STATION_ID from ", w586, " Where PLAN_DATE between '%s' and '%s' and STATION_ID='%s'") -> (w585:string)
            n107 = Format Into String(format string=w585, w576, w575, w574) -> (resulting string=w573:string)  [unwired: 2 in, 1 out]
            n108 = call "Execute query.vi"("error in (no error)"=w580, "String"=w573, "connection reference"=w581) -> ("error out"=w579:errorcluster, "Table"=w583:string[][], "connection reference 2"=w587:T1)  [unwired: 3 in, 3 out]
            n109 = Build Array (concatenate)(w584, w583) -> (w582:string[][])
          }
        }
        frame "1" {
          n110 = for {
            tunnel: w599 -> [w602]
            tunnel: w598 -> [w603]
            tunnel: w595 -> [w613]
            tunnel: w594 -> [w612] mode=indexing
            shift-right: [w614] -> w596
            shift-left: w597 -> [w615]
            shift-right: [w607] -> w592
            shift-left: string[][] [] ("data") -> [w609]
            tunnel: [w606] -> w591
            tunnel: w590 -> [w605]
            tunnel: w589 -> [w601]
            tunnel: [w600] -> w588 mode=indexing
            n111 = Concatenate Strings("Select DISTINCT PLAN_DATE,REJECTION_COUNT,STATION_ID from ", w612, " Where PLAN_DATE between '%s' and '%s' and SHIFT='%s' and STATION_ID ='%s'") -> (w610:string)
            n112 = Format Into String(format string=w610, w603, w602, w613, w601) -> (resulting string=w600:string)  [unwired: 2 in, 1 out]
            n113 = call "Execute query.vi"("error in (no error)"=w605, "String"=w600, "connection reference"=w615) -> ("error out"=w606:errorcluster, "Table"=w608:string[][], "connection reference 2"=w614:T1)  [unwired: 3 in, 3 out]
            n114 = Build Array (concatenate)(w609, w608) -> (w607:string[][])
          }
        }
        frame "2" {
          n115 = for {
            tunnel: w627 -> [w630]
            tunnel: w626 -> [w631]
            tunnel: w623 -> [w641]
            tunnel: w622 -> [w640] mode=indexing
            shift-right: [w642] -> w624
            shift-left: w625 -> [w643]
            shift-right: [w635] -> w620
            shift-left: string[][] [] ("data") -> [w637]
            tunnel: [w634] -> w619
            tunnel: w618 -> [w633]
            tunnel: w617 -> [w629]
            tunnel: [w628] -> w616 mode=indexing
            n116 = Concatenate Strings("Select DISTINCT PLAN_DATE,REJECTION_COUNT,STATION_ID from ", w640, " Where PLAN_DATE between '%s' and '%s' and SHIFT='%s' and STATION_ID ='%s'") -> (w638:string)
            n117 = Format Into String(format string=w638, w631, w630, w641, w629) -> (resulting string=w628:string)  [unwired: 2 in, 1 out]
            n118 = call "Execute query.vi"("error in (no error)"=w633, "String"=w628, "connection reference"=w643) -> ("error out"=w634:errorcluster, "Table"=w636:string[][], "connection reference 2"=w642:T1)  [unwired: 3 in, 3 out]
            n119 = Build Array (concatenate)(w637, w636) -> (w635:string[][])
          }
        }
        frame "3" {
          n120 = for {
            tunnel: w655 -> [w658]
            tunnel: w654 -> [w659]
            tunnel: w651 -> [w669]
            tunnel: w650 -> [w668] mode=indexing
            shift-right: [w670] -> w652
            shift-left: w653 -> [w671]
            shift-right: [w663] -> w648
            shift-left: string[][] [] ("data") -> [w665]
            tunnel: [w662] -> w647
            tunnel: w646 -> [w661]
            tunnel: w645 -> [w657]
            tunnel: [w656] -> w644 mode=indexing
            n121 = Concatenate Strings("Select DISTINCT PLAN_DATE,REJECTION_COUNT,STATION_ID from ", w668, " Where PLAN_DATE between '%s' and '%s' and SHIFT='%s' and STATION_ID ='%s'") -> (w666:string)
            n122 = Format Into String(format string=w666, w659, w658, w669, w657) -> (resulting string=w656:string)  [unwired: 2 in, 1 out]
            n123 = call "Execute query.vi"("error in (no error)"=w661, "String"=w656, "connection reference"=w671) -> ("error out"=w662:errorcluster, "Table"=w664:string[][], "connection reference 2"=w670:T1)  [unwired: 3 in, 3 out]
            n124 = Build Array (concatenate)(w665, w664) -> (w663:string[][])
          }
        }
      }
    }
    frame "ST 4" {
      n125 = case shown="\"ALL\", Default" w683 {
        selector: w683 -> [w691 w718 w746 w774]
        tunnel: w682 -> [w695 w722 w750 w778]
        tunnel: w681 -> [w694 w721 w749 w777]
        tunnel: w680 -> [_ _ _ _]
        tunnel: [w688 w715 w743 w771] -> w679
        tunnel: w678 -> [w693 w720 w748 w776]
        tunnel: [w692 w719 w747 w775] -> w677
        tunnel: w676 -> [w690 w717 w745 w773]
        tunnel: w675 -> [w687 w713 w741 w769]
        tunnel: [w686 w714 w742 w770] -> w674
        tunnel: "4" -> [w685 w712 w740 w768]
        tunnel: [w684 w711 w739 w767] -> w672
        frame "ALL", Default {
          n126 = for {
            tunnel: w695 -> [w698]
            tunnel: w694 -> [w699]
            tunnel: w691 -> [_]
            tunnel: w690 -> [w709] mode=indexing
            shift-right: [w710] -> w692
            shift-left: w693 -> [w704]
            shift-right: [w705] -> w688
            shift-left: string[][] [] ("data") -> [w707]
            tunnel: w687 -> [w703]
            tunnel: [w702] -> w686
            tunnel: w685 -> [w697]
            tunnel: [w696] -> w684 mode=indexing
            n127 = Concatenate Strings("Select DISTINCT PLAN_DATE,REJECTION_COUNT,STATION_ID from ", w709, " Where PLAN_DATE between '%s' and '%s' and STATION_ID='%s'") -> (w708:string)
            n128 = Format Into String(format string=w708, w699, w698, w697) -> (resulting string=w696:string)  [unwired: 2 in, 1 out]
            n129 = call "Execute query.vi"("error in (no error)"=w703, "String"=w696, "connection reference"=w704) -> ("error out"=w702:errorcluster, "Table"=w706:string[][], "connection reference 2"=w710:T1)  [unwired: 3 in, 3 out]
            n130 = Build Array (concatenate)(w707, w706) -> (w705:string[][])
          }
        }
        frame "1" {
          n131 = for {
            tunnel: w722 -> [w725]
            tunnel: w721 -> [w726]
            tunnel: w718 -> [w736]
            tunnel: w717 -> [w735] mode=indexing
            shift-right: [w737] -> w719
            shift-left: w720 -> [w738]
            shift-right: [w730] -> w715
            shift-left: string[][] [] ("data") -> [w732]
            tunnel: [w729] -> w714
            tunnel: w713 -> [w728]
            tunnel: w712 -> [w724]
            tunnel: [w723] -> w711 mode=indexing
            n132 = Concatenate Strings("Select DISTINCT PLAN_DATE,REJECTION_COUNT,STATION_ID from ", w735, " Where PLAN_DATE between '%s' and '%s' and SHIFT='%s' and STATION_ID ='%s'") -> (w733:string)
            n133 = Format Into String(format string=w733, w726, w725, w736, w724) -> (resulting string=w723:string)  [unwired: 2 in, 1 out]
            n134 = call "Execute query.vi"("error in (no error)"=w728, "String"=w723, "connection reference"=w738) -> ("error out"=w729:errorcluster, "Table"=w731:string[][], "connection reference 2"=w737:T1)  [unwired: 3 in, 3 out]
            n135 = Build Array (concatenate)(w732, w731) -> (w730:string[][])
          }
        }
        frame "2" {
          n136 = for {
            tunnel: w750 -> [w753]
            tunnel: w749 -> [w754]
            tunnel: w746 -> [w764]
            tunnel: w745 -> [w763] mode=indexing
            shift-right: [w765] -> w747
            shift-left: w748 -> [w766]
            shift-right: [w758] -> w743
            shift-left: string[][] [] ("data") -> [w760]
            tunnel: [w757] -> w742
            tunnel: w741 -> [w756]
            tunnel: w740 -> [w752]
            tunnel: [w751] -> w739 mode=indexing
            n137 = Concatenate Strings("Select DISTINCT PLAN_DATE,REJECTION_COUNT,STATION_ID from ", w763, " Where PLAN_DATE between '%s' and '%s' and SHIFT='%s' and STATION_ID ='%s'") -> (w761:string)
            n138 = Format Into String(format string=w761, w754, w753, w764, w752) -> (resulting string=w751:string)  [unwired: 2 in, 1 out]
            n139 = call "Execute query.vi"("error in (no error)"=w756, "String"=w751, "connection reference"=w766) -> ("error out"=w757:errorcluster, "Table"=w759:string[][], "connection reference 2"=w765:T1)  [unwired: 3 in, 3 out]
            n140 = Build Array (concatenate)(w760, w759) -> (w758:string[][])
          }
        }
        frame "3" {
          n141 = for {
            tunnel: w778 -> [w781]
            tunnel: w777 -> [w782]
            tunnel: w774 -> [w792]
            tunnel: w773 -> [w791] mode=indexing
            shift-right: [w793] -> w775
            shift-left: w776 -> [w794]
            shift-right: [w786] -> w771
            shift-left: string[][] [] ("data") -> [w788]
            tunnel: [w785] -> w770
            tunnel: w769 -> [w784]
            tunnel: w768 -> [w780]
            tunnel: [w779] -> w767 mode=indexing
            n142 = Concatenate Strings("Select DISTINCT PLAN_DATE,REJECTION_COUNT,STATION_ID from ", w791, " Where PLAN_DATE between '%s' and '%s' and SHIFT='%s' and STATION_ID ='%s'") -> (w789:string)
            n143 = Format Into String(format string=w789, w782, w781, w792, w780) -> (resulting string=w779:string)  [unwired: 2 in, 1 out]
            n144 = call "Execute query.vi"("error in (no error)"=w784, "String"=w779, "connection reference"=w794) -> ("error out"=w785:errorcluster, "Table"=w787:string[][], "connection reference 2"=w793:T1)  [unwired: 3 in, 3 out]
            n145 = Build Array (concatenate)(w788, w787) -> (w786:string[][])
          }
        }
      }
    }
    frame "ST 5" {
      n146 = case shown="\"ALL\", Default" w806 {
        selector: w806 -> [w814 w841 w869 w897]
        tunnel: w805 -> [w818 w845 w873 w901]
        tunnel: w804 -> [w817 w844 w872 w900]
        tunnel: w803 -> [_ _ _ _]
        tunnel: [w811 w838 w866 w894] -> w802
        tunnel: w801 -> [w816 w843 w871 w899]
        tunnel: [w815 w842 w870 w898] -> w800
        tunnel: w799 -> [w813 w840 w868 w896]
        tunnel: w798 -> [w810 w836 w864 w892]
        tunnel: [w809 w837 w865 w893] -> w797
        tunnel: "5" -> [w808 w835 w863 w891]
        tunnel: [w807 w834 w862 w890] -> w795
        frame "ALL", Default {
          n147 = for {
            tunnel: w818 -> [w821]
            tunnel: w817 -> [w822]
            tunnel: w814 -> [_]
            tunnel: w813 -> [w832] mode=indexing
            shift-right: [w833] -> w815
            shift-left: w816 -> [w827]
            shift-right: [w828] -> w811
            shift-left: string[][] [] ("data") -> [w830]
            tunnel: w810 -> [w826]
            tunnel: [w825] -> w809
            tunnel: w808 -> [w820]
            tunnel: [w819] -> w807 mode=indexing
            n148 = Concatenate Strings("Select DISTINCT PLAN_DATE,REJECTION_COUNT,STATION_ID from ", w832, " Where PLAN_DATE between '%s' and '%s' and STATION_ID='%s'") -> (w831:string)
            n149 = Format Into String(format string=w831, w822, w821, w820) -> (resulting string=w819:string)  [unwired: 2 in, 1 out]
            n150 = call "Execute query.vi"("error in (no error)"=w826, "String"=w819, "connection reference"=w827) -> ("error out"=w825:errorcluster, "Table"=w829:string[][], "connection reference 2"=w833:T1)  [unwired: 3 in, 3 out]
            n151 = Build Array (concatenate)(w830, w829) -> (w828:string[][])
          }
        }
        frame "1" {
          n152 = for {
            tunnel: w845 -> [w848]
            tunnel: w844 -> [w849]
            tunnel: w841 -> [w859]
            tunnel: w840 -> [w858] mode=indexing
            shift-right: [w860] -> w842
            shift-left: w843 -> [w861]
            shift-right: [w853] -> w838
            shift-left: string[][] [] ("data") -> [w855]
            tunnel: [w852] -> w837
            tunnel: w836 -> [w851]
            tunnel: w835 -> [w847]
            tunnel: [w846] -> w834 mode=indexing
            n153 = Concatenate Strings("Select DISTINCT PLAN_DATE,REJECTION_COUNT,STATION_ID from ", w858, " Where PLAN_DATE between '%s' and '%s' and SHIFT='%s' and STATION_ID ='%s'") -> (w856:string)
            n154 = Format Into String(format string=w856, w849, w848, w859, w847) -> (resulting string=w846:string)  [unwired: 2 in, 1 out]
            n155 = call "Execute query.vi"("error in (no error)"=w851, "String"=w846, "connection reference"=w861) -> ("error out"=w852:errorcluster, "Table"=w854:string[][], "connection reference 2"=w860:T1)  [unwired: 3 in, 3 out]
            n156 = Build Array (concatenate)(w855, w854) -> (w853:string[][])
          }
        }
        frame "2" {
          n157 = for {
            tunnel: w873 -> [w876]
            tunnel: w872 -> [w877]
            tunnel: w869 -> [w887]
            tunnel: w868 -> [w886] mode=indexing
            shift-right: [w888] -> w870
            shift-left: w871 -> [w889]
            shift-right: [w881] -> w866
            shift-left: string[][] [] ("data") -> [w883]
            tunnel: [w880] -> w865
            tunnel: w864 -> [w879]
            tunnel: w863 -> [w875]
            tunnel: [w874] -> w862 mode=indexing
            n158 = Concatenate Strings("Select DISTINCT PLAN_DATE,REJECTION_COUNT,STATION_ID from ", w886, " Where PLAN_DATE between '%s' and '%s' and SHIFT='%s' and STATION_ID ='%s'") -> (w884:string)
            n159 = Format Into String(format string=w884, w877, w876, w887, w875) -> (resulting string=w874:string)  [unwired: 2 in, 1 out]
            n160 = call "Execute query.vi"("error in (no error)"=w879, "String"=w874, "connection reference"=w889) -> ("error out"=w880:errorcluster, "Table"=w882:string[][], "connection reference 2"=w888:T1)  [unwired: 3 in, 3 out]
            n161 = Build Array (concatenate)(w883, w882) -> (w881:string[][])
          }
        }
        frame "3" {
          n162 = for {
            tunnel: w901 -> [w904]
            tunnel: w900 -> [w905]
            tunnel: w897 -> [w915]
            tunnel: w896 -> [w914] mode=indexing
            shift-right: [w916] -> w898
            shift-left: w899 -> [w917]
            shift-right: [w909] -> w894
            shift-left: string[][] [] ("data") -> [w911]
            tunnel: [w908] -> w893
            tunnel: w892 -> [w907]
            tunnel: w891 -> [w903]
            tunnel: [w902] -> w890 mode=indexing
            n163 = Concatenate Strings("Select DISTINCT PLAN_DATE,REJECTION_COUNT,STATION_ID from ", w914, " Where PLAN_DATE between '%s' and '%s' and SHIFT='%s' and STATION_ID ='%s'") -> (w912:string)
            n164 = Format Into String(format string=w912, w905, w904, w915, w903) -> (resulting string=w902:string)  [unwired: 2 in, 1 out]
            n165 = call "Execute query.vi"("error in (no error)"=w907, "String"=w902, "connection reference"=w917) -> ("error out"=w908:errorcluster, "Table"=w910:string[][], "connection reference 2"=w916:T1)  [unwired: 3 in, 3 out]
            n166 = Build Array (concatenate)(w911, w910) -> (w909:string[][])
          }
        }
      }
    }
    frame "ST 6" {
      n167 = case shown="\"ALL\", Default" w929 {
        selector: w929 -> [w937 w964 w992 w1020]
        tunnel: w928 -> [w941 w968 w996 w1024]
        tunnel: w927 -> [w940 w967 w995 w1023]
        tunnel: w926 -> [_ _ _ _]
        tunnel: [w934 w961 w989 w1017] -> w925
        tunnel: w924 -> [w939 w966 w994 w1022]
        tunnel: [w938 w965 w993 w1021] -> w923
        tunnel: w922 -> [w936 w963 w991 w1019]
        tunnel: w921 -> [w933 w959 w987 w1015]
        tunnel: [w932 w960 w988 w1016] -> w920
        tunnel: "6" -> [w931 w958 w986 w1014]
        tunnel: [w930 w957 w985 w1013] -> w918
        frame "ALL", Default {
          n168 = for {
            tunnel: w941 -> [w944]
            tunnel: w940 -> [w945]
            tunnel: w937 -> [_]
            tunnel: w936 -> [w955] mode=indexing
            shift-right: [w956] -> w938
            shift-left: w939 -> [w950]
            shift-right: [w951] -> w934
            shift-left: string[][] [] ("data") -> [w953]
            tunnel: w933 -> [w949]
            tunnel: [w948] -> w932
            tunnel: w931 -> [w943]
            tunnel: [w942] -> w930 mode=indexing
            n169 = Concatenate Strings("Select DISTINCT PLAN_DATE,REJECTION_COUNT,STATION_ID from ", w955, " Where PLAN_DATE between '%s' and '%s' and STATION_ID='%s'") -> (w954:string)
            n170 = Format Into String(format string=w954, w945, w944, w943) -> (resulting string=w942:string)  [unwired: 2 in, 1 out]
            n171 = call "Execute query.vi"("error in (no error)"=w949, "String"=w942, "connection reference"=w950) -> ("error out"=w948:errorcluster, "Table"=w952:string[][], "connection reference 2"=w956:T1)  [unwired: 3 in, 3 out]
            n172 = Build Array (concatenate)(w953, w952) -> (w951:string[][])
          }
        }
        frame "1" {
          n173 = for {
            tunnel: w968 -> [w971]
            tunnel: w967 -> [w972]
            tunnel: w964 -> [w982]
            tunnel: w963 -> [w981] mode=indexing
            shift-right: [w983] -> w965
            shift-left: w966 -> [w984]
            shift-right: [w976] -> w961
            shift-left: string[][] [] ("data") -> [w978]
            tunnel: [w975] -> w960
            tunnel: w959 -> [w974]
            tunnel: w958 -> [w970]
            tunnel: [w969] -> w957 mode=indexing
            n174 = Concatenate Strings("Select DISTINCT PLAN_DATE,REJECTION_COUNT,STATION_ID from ", w981, " Where PLAN_DATE between '%s' and '%s' and SHIFT='%s' and STATION_ID ='%s'") -> (w979:string)
            n175 = Format Into String(format string=w979, w972, w971, w982, w970) -> (resulting string=w969:string)  [unwired: 2 in, 1 out]
            n176 = call "Execute query.vi"("error in (no error)"=w974, "String"=w969, "connection reference"=w984) -> ("error out"=w975:errorcluster, "Table"=w977:string[][], "connection reference 2"=w983:T1)  [unwired: 3 in, 3 out]
            n177 = Build Array (concatenate)(w978, w977) -> (w976:string[][])
          }
        }
        frame "2" {
          n178 = for {
            tunnel: w996 -> [w999]
            tunnel: w995 -> [w1000]
            tunnel: w992 -> [w1010]
            tunnel: w991 -> [w1009] mode=indexing
            shift-right: [w1011] -> w993
            shift-left: w994 -> [w1012]
            shift-right: [w1004] -> w989
            shift-left: string[][] [] ("data") -> [w1006]
            tunnel: [w1003] -> w988
            tunnel: w987 -> [w1002]
            tunnel: w986 -> [w998]
            tunnel: [w997] -> w985 mode=indexing
            n179 = Concatenate Strings("Select DISTINCT PLAN_DATE,REJECTION_COUNT,STATION_ID from ", w1009, " Where PLAN_DATE between '%s' and '%s' and SHIFT='%s' and STATION_ID ='%s'") -> (w1007:string)
            n180 = Format Into String(format string=w1007, w1000, w999, w1010, w998) -> (resulting string=w997:string)  [unwired: 2 in, 1 out]
            n181 = call "Execute query.vi"("error in (no error)"=w1002, "String"=w997, "connection reference"=w1012) -> ("error out"=w1003:errorcluster, "Table"=w1005:string[][], "connection reference 2"=w1011:T1)  [unwired: 3 in, 3 out]
            n182 = Build Array (concatenate)(w1006, w1005) -> (w1004:string[][])
          }
        }
        frame "3" {
          n183 = for {
            tunnel: w1024 -> [w1027]
            tunnel: w1023 -> [w1028]
            tunnel: w1020 -> [w1038]
            tunnel: w1019 -> [w1037] mode=indexing
            shift-right: [w1039] -> w1021
            shift-left: w1022 -> [w1040]
            shift-right: [w1032] -> w1017
            shift-left: string[][] [] ("data") -> [w1034]
            tunnel: [w1031] -> w1016
            tunnel: w1015 -> [w1030]
            tunnel: w1014 -> [w1026]
            tunnel: [w1025] -> w1013 mode=indexing
            n184 = Concatenate Strings("Select DISTINCT PLAN_DATE,REJECTION_COUNT,STATION_ID from ", w1037, " Where PLAN_DATE between '%s' and '%s' and SHIFT='%s' and STATION_ID ='%s'") -> (w1035:string)
            n185 = Format Into String(format string=w1035, w1028, w1027, w1038, w1026) -> (resulting string=w1025:string)  [unwired: 2 in, 1 out]
            n186 = call "Execute query.vi"("error in (no error)"=w1030, "String"=w1025, "connection reference"=w1040) -> ("error out"=w1031:errorcluster, "Table"=w1033:string[][], "connection reference 2"=w1039:T1)  [unwired: 3 in, 3 out]
            n187 = Build Array (concatenate)(w1034, w1033) -> (w1032:string[][])
          }
        }
      }
    }
  }
  "Refnum out" <- w24
  "error out" <- w12
  "all station" <- w8
  "Array" <- w3
  n188 = for {
    tunnel: w2 -> [w1042] mode=indexing
    tunnel: [w1042] -> w1 mode=indexing if=w1041
    n189 = Index Array(array=w1042, index=1) -> (element=w1044:string)
    n190 = Not Equal?(x=w1044, y="0") -> (x != y?=w1041:bool)
  }
  "Table" <- w1
  n191 = Index Array(array=w1, index (col)=0 ("disabled index (col)")) -> (element=w21:string[])  [unwired: 1 in]
  n192 = call "Search_1d_array_element.vi"("Count in"=string[] [] ("Count"), "BD Date"=w21, "Elements Found in"=string[] [] ("Elements Found")) -> ("Count out"=w11:string[], "Elements Found out"=w18:string[])  [unwired: 4 in, 1 out]
  "Elements Found out" <- w18
  "PROD_COUNT TEST" <- w11
  n193 = call "Production_count_sum.vi"("PROD_COUNT"=w11, "Table 3"=w1, "date count"=w11, "Founded dates"=w18) -> ("sum"=→"sum":i32[], "Array 3"=→"Array 3":string[][])  [unwired: 6 in]
